vi "HDF5_Init10Hz.vi"(8 "error in (no error)":errorcluster, 10 "TimeStamp":dbl, 11 "FileRef":T2 format="%.0x") -> (0 "error out":errorcluster, 2 "Invalid":bool, 3 "10HzRef":T1 {"FileRef" format="%.0x"; "84Co_dset" format="%.0x"; "72Co_dset" format="%.0x"})   [LabVIEW 2018]
uses:
  <vilib>/addons/h5labview2/base/hid_t.ctl
  Controls/Clusts/HDF5_10HzRefs.ctl
  <vilib>/addons/h5labview2/base/lib_path.vi
  <vilib>/addons/h5labview2/base/H5Equery.vi
  HDF5/lib_path_mod_20200519.vi
  <vilib>/addons/h5labview2/attrib/H5Awrite.llb/H5Awrite.xnode
  <vilib>/addons/h5labview2/group/H5G.lvlib
  <vilib>/addons/h5labview2/dataset/H5D.lvlib
panel:
  out "ChannelsInit'd":i32
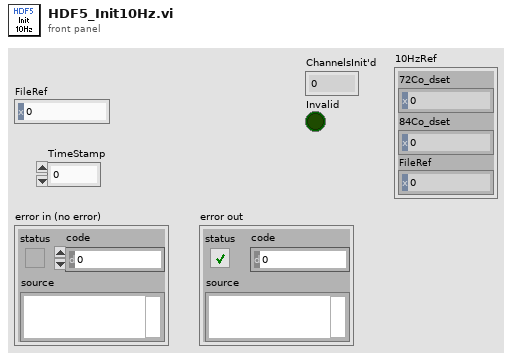
[diagram p1: front panel]
types:
  T1 = typedef "HDF5_10HzRefs.ctl" = cluster{"72Co_dset":T2, "84Co_dset":T2, "FileRef":T2}
  T2 = typedef "hid_t.ctl" = i32
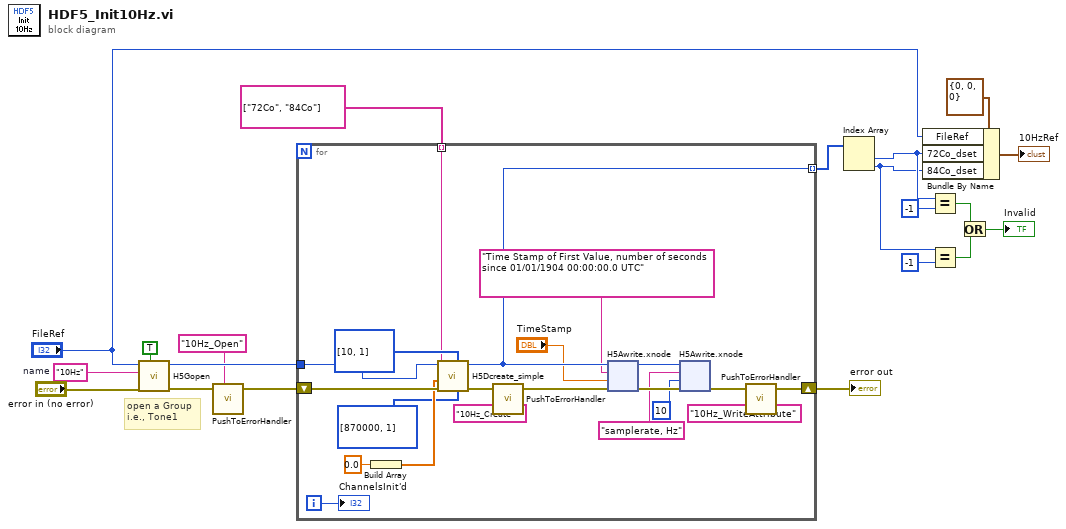
[diagram p0: block diagram]
diagram:
  w16 = "10Hz"  # name
  # "open a Group\ni.e., Tone1"
  n1 = call <vilib>:"H5Gopen.vi"("create? (F)"=TRUE, "error in (no error)"="error in (no error)", "name"=w16, "ref in"="FileRef") -> ("error out"=w12:errorcluster, "group out"=w15:T2)  [unwired: 6 in]
  n2 = call "PushToErrorHandler.vi"("ErrorIn"=w12, "ErrorLocation"="10Hz_Open") -> ("ErrorOut"=w11:errorcluster)  [unwired: 5 in]
  n3 = for {
    tunnel: w15 -> [w37]
    tunnel: string[] ["72Co", "84Co"] ("name") -> [w36] mode=indexing
    shift-right: [w22] -> w19
    shift-left: w11 -> [w41]
    tunnel: [w35] -> w20 mode=indexing
    i -> [w21]
    n4 = Build Array(sgl 0.0) -> (w40:sgl[])
    n5 = call <vilib>:"H5Dcreate_simple.vi"("max size"=u64[] [870000, 1] ("CalBeacArraySize"), "chunk size"=u64[] [10, 1], "error in (no error)"=w41, "type in"=w40, "name"=w36, "ref in"=w37) -> ("error out"=w26:errorcluster, "dset out"=w35:T2)  [unwired: 4 in]
    n6 = call "PushToErrorHandler.vi"("ErrorIn"=w26, "ErrorLocation"="10Hz_Create") -> ("ErrorOut"=w25:errorcluster)  [unwired: 5 in]
    n7 = xnode "H5Awrite.xnode"("error in (no error)"=w25, "data"="TimeStamp", "attrib name"="Time Stamp of First Value, number of seconds since 01/01/1904 00:00:00.0 UTC", "ref in"=w35) -> ("error out"=w33:errorcluster, "ref out"=w32:i32)  [unwired: 3 in, 1 out]
    n8 = xnode "H5Awrite.xnode"("error in (no error)"=w33, "data"=u32 10, "attrib name"="samplerate, Hz", "ref in"=w32) -> ("error out"=w23:errorcluster)  [unwired: 3 in, 2 out]
    n9 = call "PushToErrorHandler.vi"("ErrorIn"=w23, "ErrorLocation"="10Hz_WriteAttribute") -> ("ErrorOut"=w22:errorcluster)  [unwired: 5 in]
    "ChannelsInit'd" <- w21
  }
  "error out" <- w19
  n10 = Index Array(array=w20) -> (element #1=w9:T2, element #2=w6:T2)  [unwired: 2 in]
  n11 = Bundle By Name(cluster=T1 {"72Co_dset"=0, "84Co_dset"=0, "FileRef"=0} ("10HzRef 2"), "FileRef"="FileRef", "72Co_dset"=w9, "84Co_dset"=w6) -> (→"10HzRef":T1)
  n12 = Equal?(x=w9, y=T2 -1) -> (x = y?=w5:bool)
  n13 = Equal?(x=w6, y=T2 -1) -> (x = y?=w4:bool)
  n14 = Or(x=w5, y=w4) -> (x .or. y?=→"Invalid":bool)
